vi "Bridge Bias Open.vi"(8 "error in":errorcluster, 11 "bridge in":T1 {"TWM"."f-list [Hz]" format="%#_6p"}) -> (0 "error out":errorcluster, 2 "idn string":string, 3 "bridge out":T1 {"TWM"."f-list [Hz]" format="%#_6p"})   [LabVIEW 2013]
doc: "Open and initialize DC bias compensator."
uses:
  Bridge Session.ctl
  Bridge Type.ctl
  drivers/TWM client/TWM Session.ctl
  drivers/TWM client/TWM parameters.ctl
  drivers/TWM client/Meas Proc QWTB Uncertainty Mode.ctl
  Bridge Bias Session.ctl
  Bridge Bias Type.ctl
  <vilib>/Utility/error.llb/Error Cluster From Error Code.vi
  <vilib>/ErrorRing/Error Ring.xnode
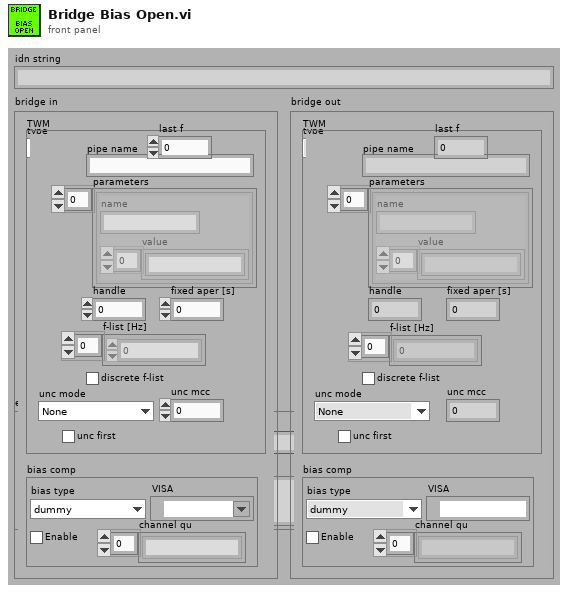
[diagram p1: front panel]
types:
  T1 = typedef "Bridge Session.ctl" = cluster{"type":T2, "TWM":T3, "last f":dbl, "bias comp":T6}
  T2 = typedef "Bridge Type.ctl" = enum16{"TWM client", "dummy"}
  T3 = typedef "TWM Session.ctl" = cluster{"pipe name":string, "parameters":T4[], "handle":i32, "fixed aper [s]":dbl, "f-list [Hz]":dbl[], "discrete f-list":bool, "unc mode":T5, "unc mcc":i32, "unc first":bool}
  T4 = typedef "TWM parameters.ctl" = cluster{"name":string, "value":string[]}
  T5 = typedef "Meas Proc QWTB Uncertainty Mode.ctl" = enum16{"None", "GUF", "Monte Carlo"}
  T6 = typedef "Bridge Bias Session.ctl" = cluster{"bias type":T7, "VISA":refnum<visa-resource-name>, "Enable":bool, "channel qu":string[]}
  T7 = typedef "Bridge Bias Type.ctl" = enum16{"dummy", "CMI LiBbias V1.0"}
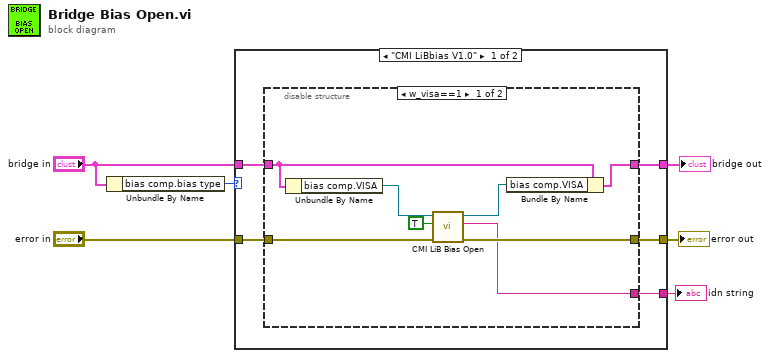
[diagram p0: block diagram]
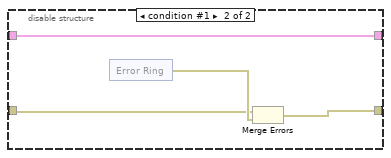
[diagram p2: hidden frame]
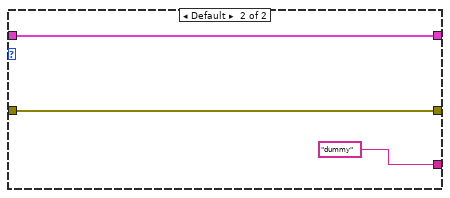
[diagram p3: hidden frame]
diagram:
  n1 = Unbundle By Name("bridge in") -> ("bias comp.bias type"=w6:T7)
  n2 = case shown="\"CMI LiBbias V1.0\"" w6 {
    tunnel: "error in" -> [w9 w31]
    tunnel: [w7 w31] -> w4
    tunnel: "bridge in" -> [w11 w30]
    tunnel: [w10 w30] -> w2
    tunnel: [w8 "dummy"] -> w1
    frame "CMI LiBbias V1.0" {
      n3 = disable-structure shown="w_visa==1" {
        disable-tunnel: w11 -> [w19 w20]
        disable-tunnel: [w18 w20] -> w10
        disable-tunnel: w9 -> [w17 w22]
        disable-tunnel: [w16 w21] -> w7
        disable-tunnel: [w13 _] -> w8
        frame condition #0 (active) {
          n4 = Unbundle By Name(w19) -> ("bias comp.VISA"=w15:refnum<visa-resource-name>)
          n5 = call "CMI LiB Bias Open.vi"("error in"=w17, "reset (false)"=TRUE, "VISA in"=w15) -> ("error out"=w16:errorcluster, "idn string"=w13:string, "VISA out"=w14:refnum<visa-resource-name>)  [unwired: 6 in]
          n6 = Bundle By Name(cluster=w19, "bias comp.VISA"=w14) -> (w18:T1)
        }
        frame condition #1 {
          n7 = xnode "Error Ring"() -> ("error out"=w23:errorcluster)
          n8 = Merge Errors(w22, w23) -> (w21:errorcluster)
        }
      }
    }
    frame Default {
    }
  }
  "error out" <- w4
  "bridge out" <- w2
  "idn string" <- w1
